vi "Configure Heater.vi"(0 "VISA resource name":refnum<visa-resource-name>, 1 "Max User Current (0.45)":dbl=0.45 min=0.0 max=0.63 step=0.001, 2 "Current Power (1: Current)":u16(ring)=1 items=["Current"=1, "Power"=2], 5 "Output (0: Sample Heater)":u16(ring) items=["Sample Heater", "Warm-up Heater (output 1)"], 7 "Heater Resistance Load (50 ohms)":i32=50 min=1 max=2000 step=1, 9 "Max Current (1: 0.45A/5W/10W)":u16(ring)=1 items=["User Specified", "0.45A/5W/10W", "0.63A/10W"], 11 "error in (no error)":errorcluster) -> (4 "VISA resource name out":refnum<visa-resource-name>, 15 "error out":errorcluster)   [LabVIEW 2019, in "Lake Shore 372.lvlib"]
doc: "Configures the heater output parameters."
uses:
  Lake Shore 372.lvlib
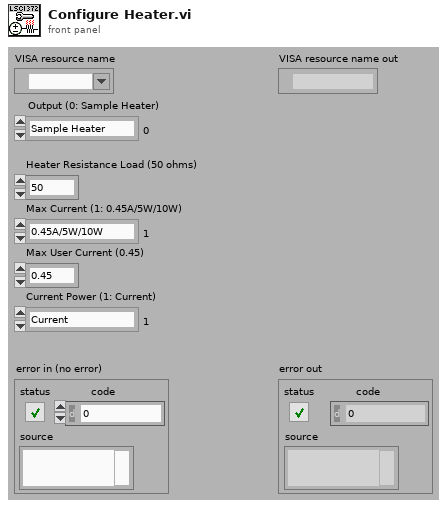
[diagram p1: front panel]
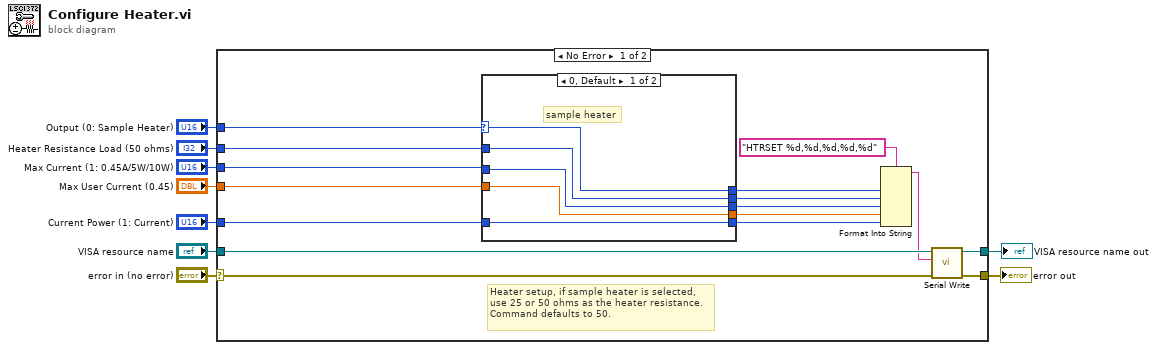
[diagram p0: block diagram]
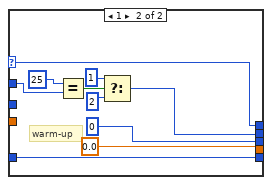
[diagram p2: hidden frame]
diagram:
  n1 = case shown="No Error" "error in (no error)" {
    selector: "error in (no error)" -> [w14 w41]
    tunnel: "VISA resource name" -> [w25 w42]
    tunnel: [w22 w42] -> w8
    tunnel: [w21 w41] -> w7
    tunnel: "Output (0: Sample Heater)" -> [w20 _]
    tunnel: "Heater Resistance Load (50 ohms)" -> [w13 _]
    tunnel: "Max Current (1: 0.45A/5W/10W)" -> [w12 _]
    tunnel: "Max User Current (0.45)" -> [w11 _]
    tunnel: "Current Power (1: Current)" -> [w10 _]
    frame No Error {
      # "Heater setup, if sample heater is selected,\nuse 25 or 50 ohms as the heater resistance.\nCommand defaults to 50."
      n2 = case shown="0, Default" w20 {
        selector: w20 -> [w28 w39]
        tunnel: w13 -> [w29 w38]
        tunnel: w12 -> [w27 _]
        tunnel: [w27 u16 0 ("Max Current")] -> w18
        tunnel: w11 -> [w26 _]
        tunnel: [w26 0.0 ("Max User Current")] -> w19
        tunnel: w10 -> [w30 w40]
        tunnel: [w30 w40] -> w17
        tunnel: [w29 w33] -> w16
        tunnel: [w28 w39] -> w15
        frame 0, Default {
          # "sample heater"
        }
        frame 1 {
          # "warm-up"
          n3 = Equal?(x=25, y=w38) -> (x = y?=w32:bool)
          n4 = Select(t=1 ("x"), s=w32, f=2 ("x")) -> (s? t:f=w33:i32)
        }
      }
      n5 = Format Into String(format string="HTRSET %d,%d,%d,%d,%d", w15, w16, w18, w19, w17) -> (resulting string=w23:string)  [unwired: 2 in, 1 out]
      n6 = call "Serial Write.vi"("error in (no error)"=w14, "Write Buffer (\"\")"=w23, "VISA resource name"=w25) -> ("error out"=w21:errorcluster, "VISA resource name out"=w22:refnum<visa-resource-name>)  [unwired: 6 in, 1 out]
    }
    frame Error {
    }
  }
  "VISA resource name out" <- w8
  "error out" <- w7
